vi "MecaOdometry_NewDefaultPose.vi"(11 "GyroOffset":T1 {"SIN" format="%13.4f"; "COS" format="%13.4f"; "VALUE" format="%13.4f"}) -> (3 "MECA_DRIVE_ODOMETRY":T2={"POSE"={"TRANSLATION"={"X"=0.0, "Y"=0.0}, "ROTATION"={"VALUE"=0.0, "COS"=1.0, "SIN"=0.0}}, "PrevTime"=0.0, "GyroOffset"={"VALUE"=0.0, "COS"=0.0, "SIN"=0.0}, "PreviousAngle"={"VALUE"=0.0, "COS"=0.0, "SIN"=0.0}} {"PreviousAngle"."SIN" format="%13.4f"; "PreviousAngle"."COS" format="%13.4f"; "PreviousAngle"."VALUE" format="%13.4f"; "GyroOffset"."SIN" format="%13.4f"; "GyroOffset"."COS" format="%13.4f"; "GyroOffset"."VALUE" format="%13.4f"; "PrevTime" format="%13.4f"; "POSE"."ROTATION"."SIN" format="%13.4f"; "POSE"."ROTATION"."COS" format="%13.4f"; "POSE"."ROTATION"."VALUE" format="%13.4f"; "POSE"."TRANSLATION"."Y" format="%14.3f"; "POSE"."TRANSLATION"."X" format="%14.3f"})   [LabVIEW 2019, in "Trajectory_Library.lvlib"]
doc: "Constructs a MecanumDriveOdometry cluster data structure with a default pose at the origin.\n\nSubVIs for mecanum drive odometry. Odometry allows you to track the robot's position on the field over a course of a match using readings from your mecanum wheel encoders.\n\nTeams can use odometry during the autonomous period for complex tasks like path following. Furthermore, odometry can be used for latency compensation when using computer-vision systems.\n\nParameters:\n - GyroOffset - The angle reported by the gyroscope. (Rotation)\n\nReturns:\n - MecaDriveOdomentry - Data structure"
uses:
  Trajectory_Library.lvlib
  MECA_DRIVE_ODOMETRY.ctl
  POSE2D.ctl
  TRANSLATION2D.ctl
  ROTATION2D.ctl
  Rotation2d_CreateAngle.vi
  Translation2d_Create.vi
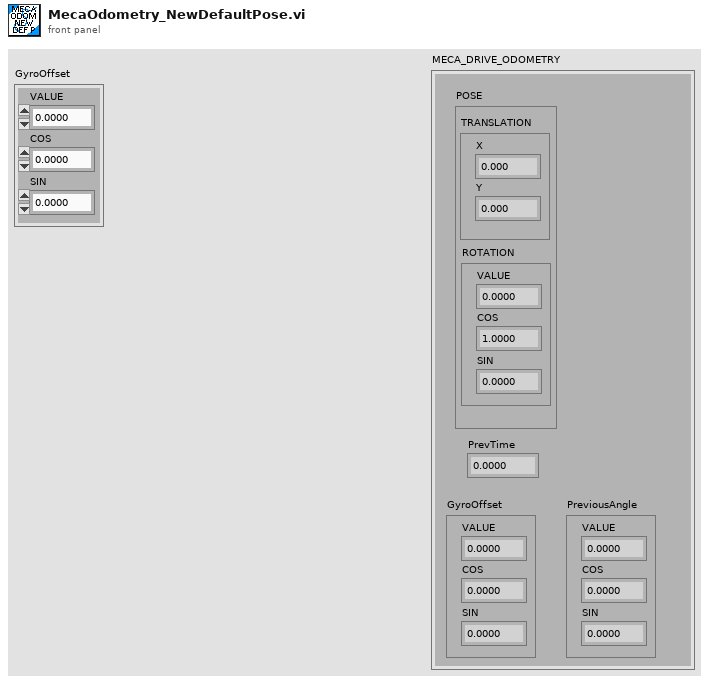
[diagram p1: front panel]
types:
  T1 = typedef "Trajectory_Library.lvlib/ROTATION2D.ctl" = cluster{"VALUE":dbl, "COS":dbl, "SIN":dbl}
  T2 = typedef "Trajectory_Library.lvlib/MECA_DRIVE_ODOMETRY.ctl" = cluster{"POSE":T3, "PrevTime":dbl, "GyroOffset":T1, "PreviousAngle":T1}
  T3 = typedef "Trajectory_Library.lvlib/POSE2D.ctl" = cluster{"TRANSLATION":T4, "ROTATION":T1}
  T4 = typedef "Trajectory_Library.lvlib/TRANSLATION2D.ctl" = cluster{"X":dbl, "Y":dbl}
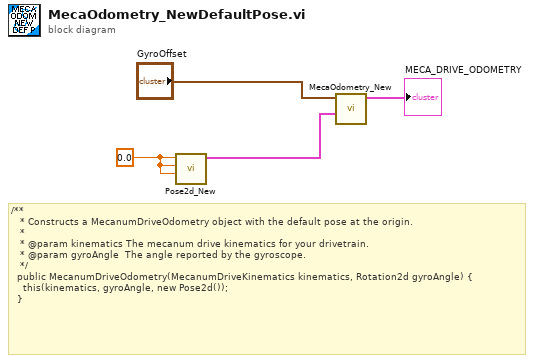
[diagram p0: block diagram]
diagram:
  w4 = 0.0 ("X")
  # "/**\n   * Constructs a MecanumDriveOdometry object with the default pose at the origin.\n   *\n   * @param kinematics The mecanum drive kinematics for your drivetrain.\n   * @param gyroAngle  The angle reported by the gyroscope.\n   */\n  public MecanumDriveOdometry(MecanumDriveKinematics kinematics, Rotation2d gyroAngle) {\n    this(kinematics, gyroAngle, new Pose2d());\n  }"
  n1 = call "Pose2d_New.vi"("Heading"=w4, "Y"=w4, "X"=w4) -> ("out POSe"=w2:T3)  [unwired: 8 in]
  n2 = call "MecaOdometry_New.vi"("POSE"=w2, "GyroOffset"="GyroOffset") -> ("MECA_DRIVE_ODOMETRY"=→"MECA_DRIVE_ODOMETRY":T2)  [unwired: 9 in]
